vi "OutputErrors.vi"(8 "errors in":errorcluster[](array[cluster]), 9 "Causing VI":string, 10 "Calling VI":string) -> (0 "error out":errorcluster)   [LabVIEW 2013]
doc: "Sends any errors that occur to the SmartDashboard. If the error, calling VI, and causing VI is identical to a previous error, the error will not be sent."
uses:
  <vilib>/Rock Robotics/Network Tables/SD Write Numeric Array.vi
  <vilib>/Rock Robotics/Network Tables/SD Write Boolean Array.vi
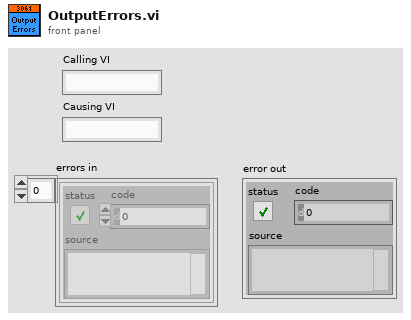
[diagram p1: front panel]
types:
  T1 = cluster{"Boolean":bool, "Numeric":i32, "String":string}
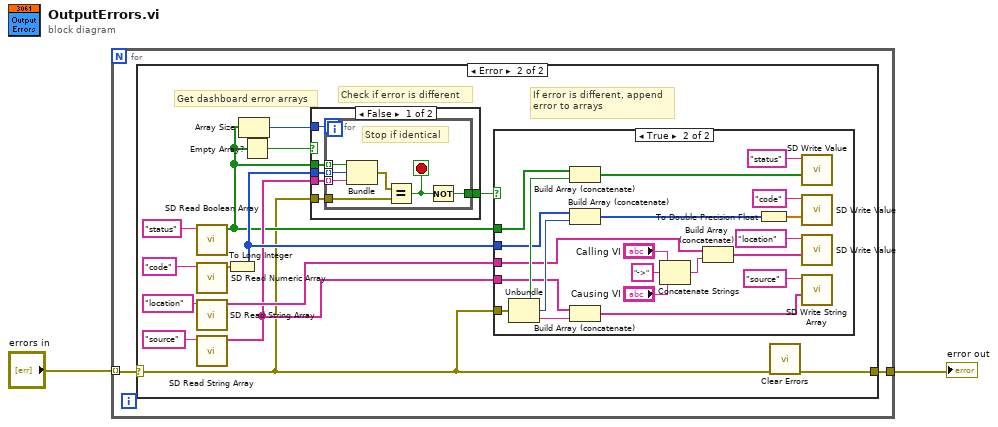
[diagram p0: block diagram]
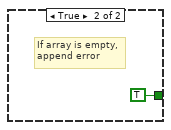
[diagram p3: hidden frame]
diagram:
  n1 = for {
    tunnel: [w4] -> w2
    tunnel: "errors in" -> [w3] mode=indexing
    n2 = case shown="Error" w3 {
      selector: w3 -> [w5 w6]
      tunnel: [w5 w7] -> w4
      frame No Error {
      }
      frame Error {
        # "Check if error is different"
        # "If error is different, append\nerror to arrays"
        # "Get dashboard error arrays"
        n3 = call <vilib>:"SD Read Boolean Array.vi"("Name"="status") -> ("Boolean Array"=w9:bool[])  [unwired: 8 in, 2 out]
        n4 = call <vilib>:"SD Read Numeric Array.vi"("Name"="code") -> ("Numeric Array"=w16:dbl[])  [unwired: 8 in, 2 out]
        n5 = call <vilib>:"SD Read String Array.vi"("Name"="location") -> ("String Array"=w12:string[])  [unwired: 9 in, 1 out]
        n6 = call <vilib>:"SD Read String Array.vi"("Name"="source") -> ("String Array"=w11:string[])  [unwired: 9 in, 1 out]
        n7 = To Long Integer(number=w16) -> (32bit integer=w14:i32[])
        n8 = Array Size(array=w9) -> (size(s)=w10:i32)
        n9 = Empty Array?(array=w9) -> (empty?=w8:bool)
        n10 = case shown="False" w8 {
          tunnel: w10 -> [w25 _]
          tunnel: w6 -> [w24 _]
          tunnel: [w23 TRUE] -> w15
          tunnel: w9 -> [w22 _]
          tunnel: w14 -> [w21 _]
          tunnel: w11 -> [w20 _]
          frame False {
            n11 = for {
              N: w25 -> [_]
              tunnel: w24 -> [w29]
              tunnel: w22 -> [w32] mode=indexing
              tunnel: w21 -> [w31] mode=indexing
              tunnel: w20 -> [w30] mode=indexing
              tunnel: [w26] -> w23
              stop <- w27 stop-if-true
              # "Stop if identical"
              n12 = Bundle("Boolean"=w32, "Numeric"=w31, "String"=w30) -> (w28:T1)  [unwired: 1 in]
              n13 = Equal?(x=w28, y=w29) -> (x = y?=w27:bool)
              n14 = Not(x=w27) -> (.not. x?=w26:bool)
            }
          }
          frame True {
            # "If array is empty,\nappend error"
          }
        }
        n15 = case shown="True" w15 {
          tunnel: w6 -> [_ w54]
          tunnel: w9 -> [_ w47]
          tunnel: w14 -> [_ w44]
          tunnel: w12 -> [_ w37]
          tunnel: w11 -> [_ w38]
          frame False {
          }
          frame True {
            n16 = Unbundle(w54) -> ("status"=w46:bool, "code"=w43:i32, "source"=w39:string)
            n17 = Build Array (concatenate)(w47, w46) -> (w45:bool[])
            n18 = Build Array (concatenate)(w44, w43) -> (w42:i32[])
            n19 = Build Array (concatenate)(w38, w39) -> (w35:string[])
            n20 = Concatenate Strings("Calling VI", "->" ("string"), "Causing VI") -> (w36:string)
            n21 = Build Array (concatenate)(w37, w36) -> (w34:string[])
            n22 = To Double Precision Float(number=w42) -> (double precision float=w41:dbl[])
            n23 = call-poly <vilib>:"SD Write Value.vi"("Boolean Array"=w45, "Name"="status") -> ()  [unwired: 8 in, 2 out]
            n24 = call-poly <vilib>:"SD Write Value.vi"("Numeric Array"=w41, "Name"="code") -> ()  [unwired: 8 in, 2 out]
            n25 = call-poly <vilib>:"SD Write Value.vi"("String Array"=w34, "Name"="location") -> ()  [unwired: 8 in, 2 out]
            n26 = call <vilib>:"SD Write String Array.vi"("String Array"=w35, "Name"="source") -> ()  [unwired: 8 in, 2 out]
          }
        }
        n27 = call <vilib>:"Clear Errors.vi"("error in (no error)"=w6) -> ("error out"=w7:errorcluster)  [unwired: 6 in]
      }
    }
  }
  "error out" <- w2
